vi "Data Write Back.vi"(8 "error in (no error)":errorcluster, 9 "Tag In":string, 10 "Tree In":refnum<class "Tree.lvclass">, 11 "Tree Data in":refnum<class "Tree Data.lvclass">) -> (0 "error out":errorcluster, 1 "Data Out":T1, 2 "Tree Out":refnum<class "Tree.lvclass">, 3 "Tree Data out":refnum<class "Tree Data.lvclass">)   [LabVIEW 2024, in "Tree Data.lvclass"]
uses:
  Tree Data.lvclass
  Tree/Tree.lvclass
  Tree/Type Def/Tree Item.ctl
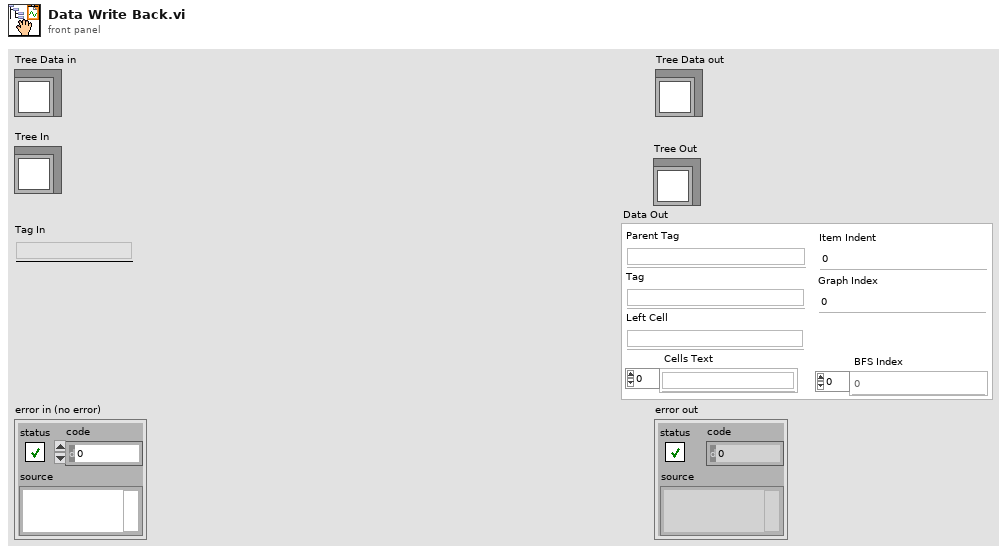
[diagram p1: front panel]
types:
  T1 = typedef "Tree Item.ctl" = cluster{"Parent Tag":string, "Tag":string, "Left Cell":string, "Cells Text":string[], "BFS Index":i32[], "Graph Index":i32, "Item Indent":i32}
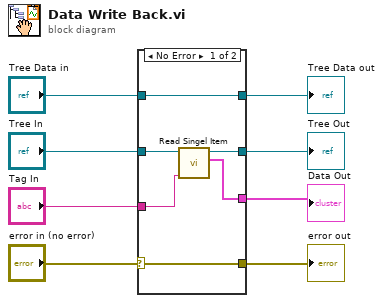
[diagram p0: block diagram]
diagram:
  n1 = case shown="No Error" "error in (no error)" {
    selector: "error in (no error)" -> [w11 w17]
    tunnel: [w11 w17] -> w7
    tunnel: [w14 w16] -> w5
    tunnel: "Tree Data in" -> [w14 w16]
    tunnel: [w12 w15] -> w4
    tunnel: "Tree In" -> [w13 w15]
    tunnel: [w10 _] -> w2
    tunnel: "Tag In" -> [w9 _]
    frame No Error {
      n2 = call "Read Singel Item.vi"("Tag"=w9, "Tree in"=w13) -> ("Element Out"=w10:T1, "Tree out"=w12:refnum<class "Tree.lvclass">)  [unwired: 8 in]
    }
    frame Error {
    }
  }
  "error out" <- w7
  "Tree Data out" <- w5
  "Tree Out" <- w4
  "Data Out" <- w2
